vi "Noyito10ChannelADC_MultiSampleAllChannels.vi"(0 "Timeout (s)":dbl=30.0, 5 "Average While Running?":bool, 7 "# of Samples":u8=30, 11 "error in (no error)":errorcluster) -> (3 "Error":bool, 4 "ADC Voltages - RT Values":T4, 6 "ADC Counts - RT Values":T3, 8 "ADC Voltages":T2(array[cluster]), 10 "ADC Counts":T1(array[cluster]), 13 "ADC Voltages - Mean Values":T4, 14 "ADC Counts - Mean Values":T3, 15 "error out":errorcluster)   [LabVIEW 2020, in "NOYITO 10 Channel ADC Module Driver.lvlib"]
uses:
  NOYITO 10 Channel ADC Module Driver.lvlib
panel:
  in  "Tab Control":enum32{"Page 1", "Page 2"}(tab)
  out "Current Sample #":i32
  out "Full Sample Text":string
  in  "STOP SAMPLING":bool
  # "*Approx. 2 samples per second"
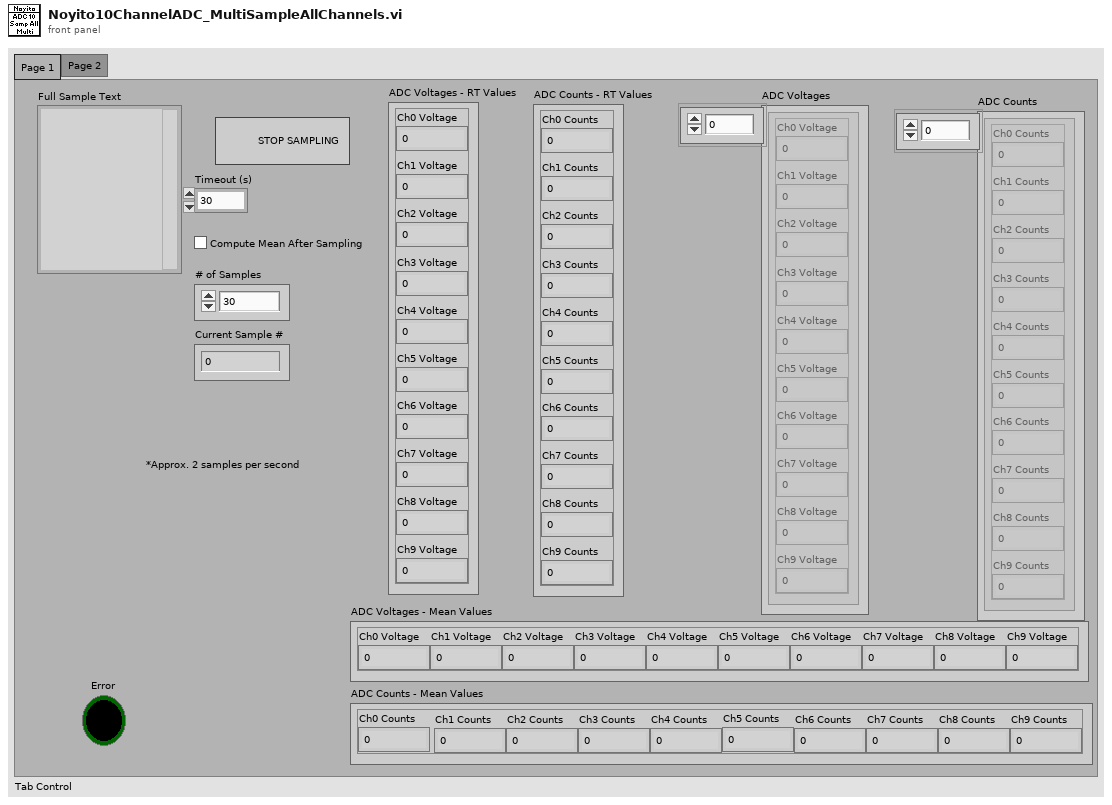
[diagram p1: front panel]
types:
  T1 = cluster{"Ch0 Counts":u16, "Ch1 Counts":u16, "Ch2 Counts":u16, "Ch3 Counts":u16, "Ch4 Counts":u16, "Ch5 Counts":u16, "Ch6 Counts":u16, "Ch7 Counts":u16, "Ch8 Counts":u16, "Ch9 Counts":u16}[]
  T2 = cluster{"Ch0 Voltage":dbl, "Ch1 Voltage":dbl, "Ch2 Voltage":dbl, "Ch3 Voltage":dbl, "Ch4 Voltage":dbl, "Ch5 Voltage":dbl, "Ch6 Voltage":dbl, "Ch7 Voltage":dbl, "Ch8 Voltage":dbl, "Ch9 Voltage":dbl}[]
  T3 = cluster{"Ch0 Counts":u16, "Ch1 Counts":u16, "Ch2 Counts":u16, "Ch3 Counts":u16, "Ch4 Counts":u16, "Ch5 Counts":u16, "Ch6 Counts":u16, "Ch7 Counts":u16, "Ch8 Counts":u16, "Ch9 Counts":u16}
  T4 = cluster{"Ch0 Voltage":dbl, "Ch1 Voltage":dbl, "Ch2 Voltage":dbl, "Ch3 Voltage":dbl, "Ch4 Voltage":dbl, "Ch5 Voltage":dbl, "Ch6 Voltage":dbl, "Ch7 Voltage":dbl, "Ch8 Voltage":dbl, "Ch9 Voltage":dbl}
  T5 = cluster{"[0]":dbl, "[1]":dbl, "[2]":dbl, "[3]":dbl, "[4]":dbl, "[5]":dbl, "[6]":dbl, "[7]":dbl, "[8]":dbl, "[9]":dbl}
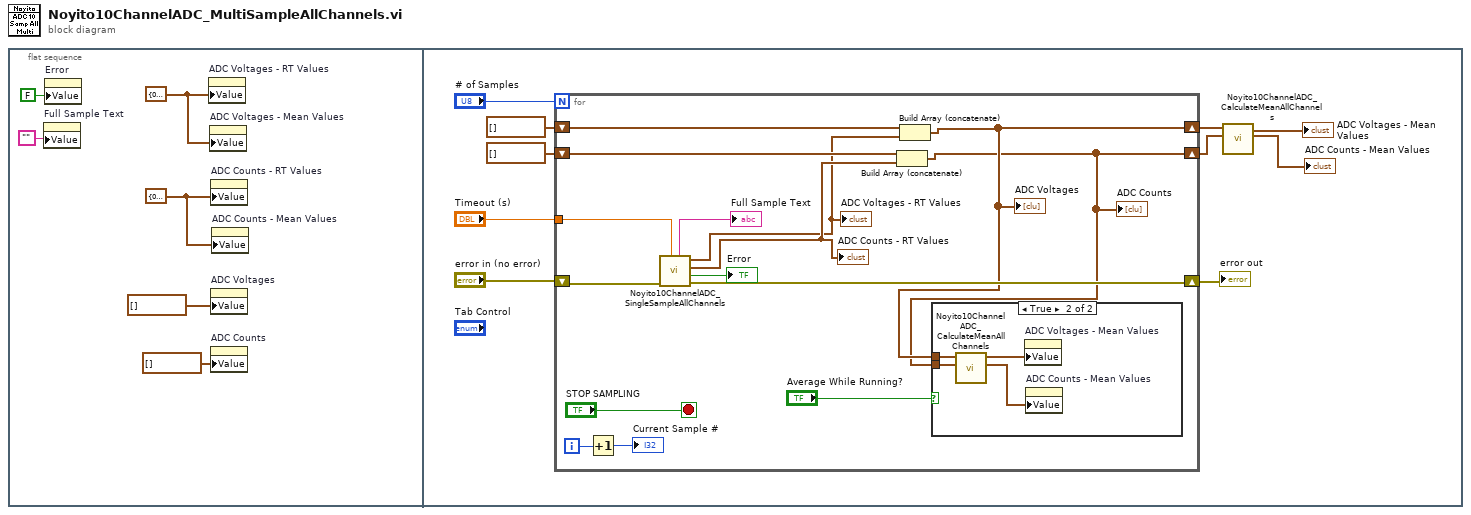
[diagram p0: block diagram]
diagram:
  n1 = flat-sequence {
    frame #0 {
      w3 = T3 {"Ch0 Counts"=0, "Ch1 Counts"=0, "Ch2 Counts"=0, "Ch3 Counts"=0, "Ch4 Counts"=0, "Ch5 Counts"=0, "Ch6 Counts"=0, "Ch7 Counts"=0, "Ch8 Counts"=0, "Ch9 Counts"=0} ("ADC Counts - RT Values")
      w4 = T4 {"Ch0 Voltage"=0.0, "Ch1 Voltage"=0.0, "Ch2 Voltage"=0.0, "Ch3 Voltage"=0.0, "Ch4 Voltage"=0.0, "Ch5 Voltage"=0.0, "Ch6 Voltage"=0.0, "Ch7 Voltage"=0.0, "Ch8 Voltage"=0.0, "Ch9 Voltage"=0.0} ("ADC Voltages - RT Values")
      n2 = property on="Full Sample Text" class="Str"("Value"="") -> ()  [unwired: 2 in, 2 out]
      n3 = property on="Error" class="Bool (strict)"("Value"=FALSE ("Error")) -> ()  [unwired: 2 in, 2 out]
      n4 = property on="ADC Voltages - RT Values" class="Clust (strict)"("Value"=w4) -> ()  [unwired: 2 in, 2 out]
      n5 = property on="ADC Voltages - Mean Values" class="Clust (strict)"("Value"=w4) -> ()  [unwired: 2 in, 2 out]
      n6 = property on="ADC Counts - RT Values" class="Clust (strict)"("Value"=w3) -> ()  [unwired: 2 in, 2 out]
      n7 = property on="ADC Voltages" class="Arr (strict)"("Value"=T2 [] ("ADC Voltages")) -> ()  [unwired: 2 in, 2 out]
      n8 = property on="ADC Counts" class="Arr (strict)"("Value"=T1 [] ("ADC Counts")) -> ()  [unwired: 2 in, 2 out]
      n9 = property on="ADC Counts - Mean Values" class="Clust (strict)"("Value"=w3) -> ()  [unwired: 2 in, 2 out]
    }
    frame #1 {
      n10 = for {
        N: "# of Samples" -> [_]
        tunnel: "Timeout (s)" -> [w31]
        shift-right: [w27] -> w13
        shift-left: "error in (no error)" -> [w28]
        shift-right: [w18] -> w9
        shift-left: T1 [] -> [w24]
        shift-right: [w19] -> w10
        shift-left: T2 [] -> [w25]
        i -> [w22]
        stop <- "STOP SAMPLING" stop-if-true
        n11 = Increment(x=w22) -> (x+1=→"Current Sample #":i32)
        n12 = call "Noyito10ChannelADC_SingleSampleAllChannels.vi"("Timeout (s)"=w31, "error in (no error)"=w28) -> ("error out"=w27:errorcluster, "Error"=→"Error":bool, "ADC Counts"=w23:T3, "ADC Voltages"=w20:T4, "Full Sample Text"=→"Full Sample Text":string)  [unwired: 5 in]
        "ADC Voltages - RT Values" <- w20
        "ADC Counts - RT Values" <- w23
        n13 = Build Array (concatenate)(w24, w23) -> (w18:T1)
        "ADC Counts" <- w18
        n14 = Build Array (concatenate)(w25, w20) -> (w19:T2)
        "ADC Voltages" <- w19
        n15 = case shown="True" "Average While Running?" {
          tunnel: w19 -> [_ w35]
          tunnel: w18 -> [_ w34]
          frame False {
          }
          frame True {
            n16 = call "Noyito10ChannelADC_CalculateMeanAllChannels.vi"("ADC Counts"=w34, "ADC Voltages"=w35) -> ("ADC Counts - Mean Values"=w32:T5, "ADC Voltages - Mean Values"=w33:T5)  [unwired: 8 in]
            n17 = property on="ADC Voltages - Mean Values" class="Clust (strict)"("Value"=w33) -> ()  [unwired: 2 in, 2 out]
            n18 = property on="ADC Counts - Mean Values" class="Clust (strict)"("Value"=w32) -> ()  [unwired: 2 in, 2 out]
          }
        }
      }
      "error out" <- w13
      n19 = call "Noyito10ChannelADC_CalculateMeanAllChannels.vi"("ADC Counts"=w9, "ADC Voltages"=w10) -> ("ADC Counts - Mean Values"=→"ADC Counts - Mean Values":T5, "ADC Voltages - Mean Values"=→"ADC Voltages - Mean Values":T5)  [unwired: 8 in]
    }
  }
